vi "Transcriptor LabVIEW to C code Translator 2.vi"(0 "Input":variant=variant("Function Name"=variant(string "Strip Path"), "Input Datatypes"=variant(string[] ["error", "int"]), "Inputs"=variant(string[] ["error in", "x"]), "Node refnum"=variant(refnum<vi> refnum), "Output Datatypes"=variant(string[] ["int"]), "Outputs"=variant(string[] ["a"])), 11 "error in (no error)":errorcluster) -> (4 "Output":variant=variant("Defines"=variant(string[] []), "Includes"=variant(string[] []), "Replaced Code"=variant(string "/* LabVIEW system function 'Strip Path' not found. */")), 15 "error out":errorcluster)   [LabVIEW 2014]
doc: "An example of how to create the Translator to convert the LabVIEW VIs to Arduino C code."
panel:
  out "Outputs":string[](array[string])
  out "Inputs":string[](array[string])
  out "Output Datatypes":string[](array[string])
  out "Input Datatypes":string[](array[string])
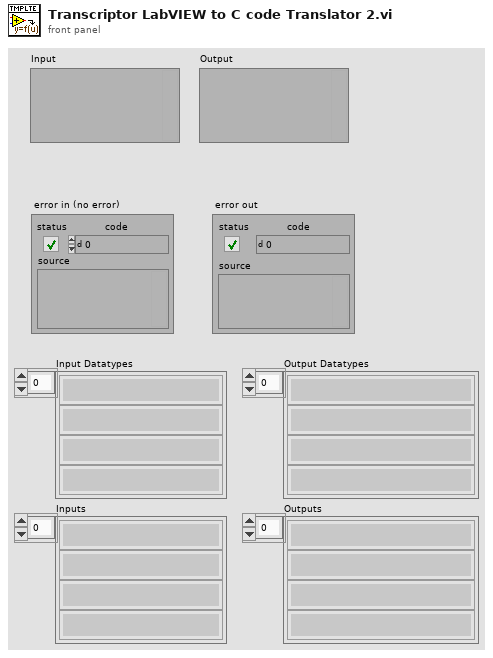
[diagram p1: front panel]
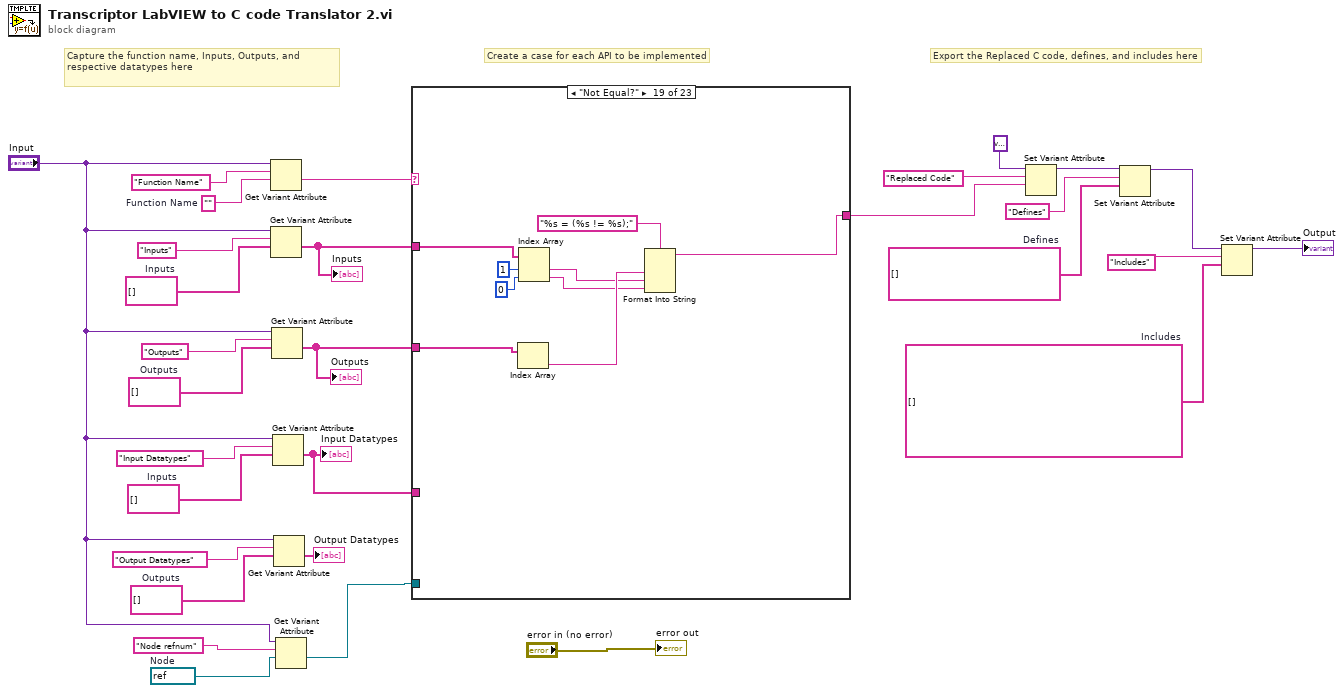
[diagram p0: block diagram]
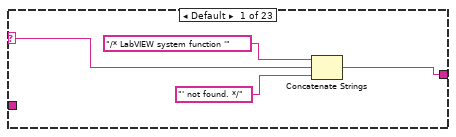
[diagram p2: hidden frame]
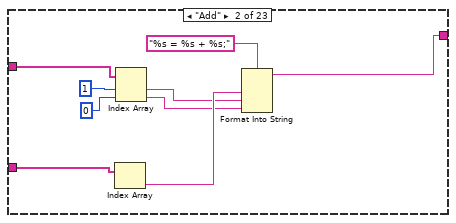
[diagram p3: hidden frame]
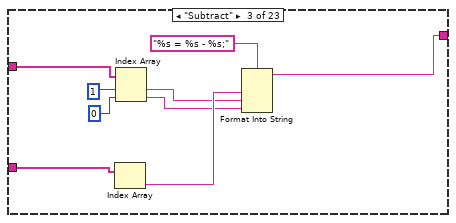
[diagram p4: hidden frame]
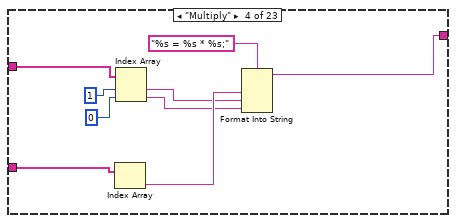
[diagram p5: hidden frame]
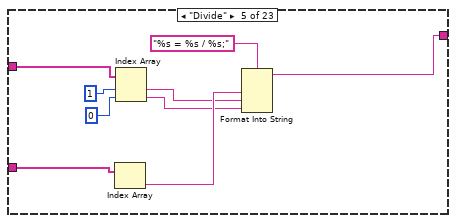
[diagram p6: hidden frame]
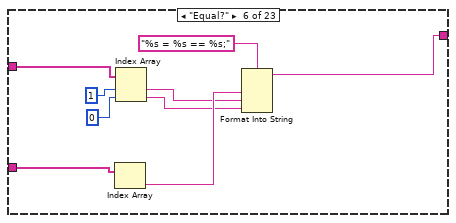
[diagram p7: hidden frame]
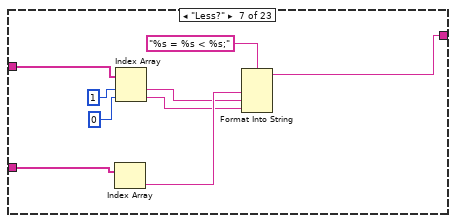
[diagram p8: hidden frame]
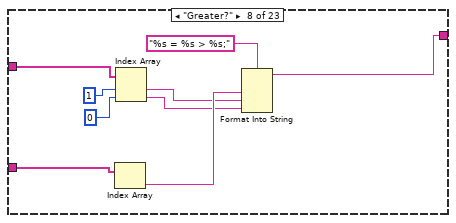
[diagram p9: hidden frame]
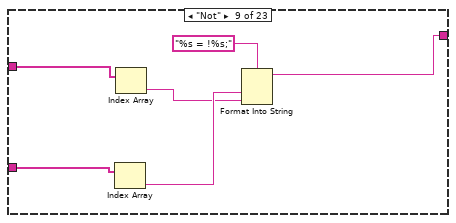
[diagram p10: hidden frame]
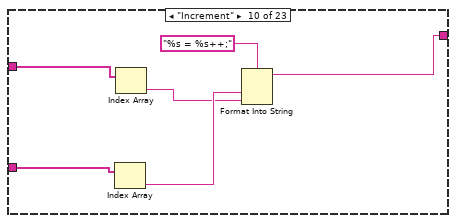
[diagram p11: hidden frame]
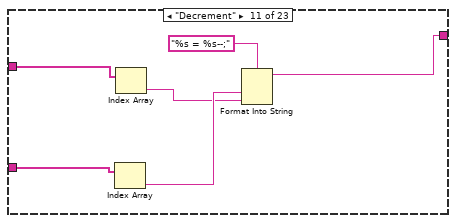
[diagram p12: hidden frame]
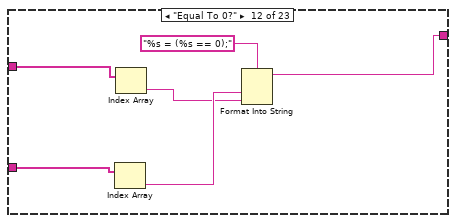
[diagram p13: hidden frame]
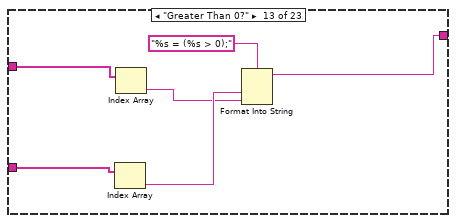
[diagram p14: hidden frame]
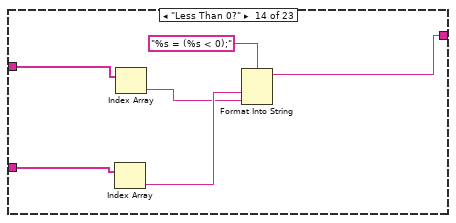
[diagram p15: hidden frame]
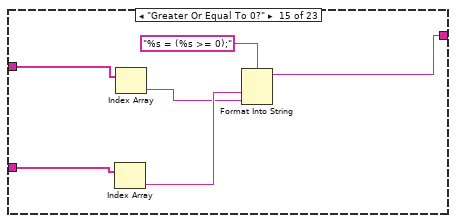
[diagram p16: hidden frame]
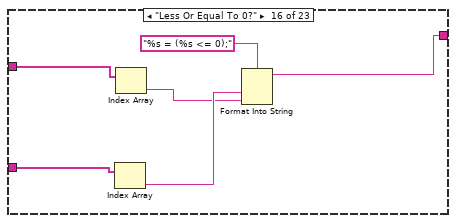
[diagram p17: hidden frame]
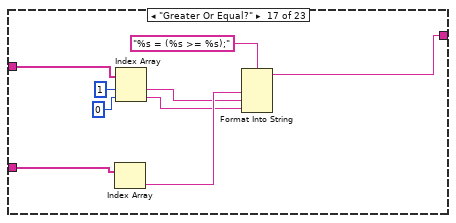
[diagram p18: hidden frame]
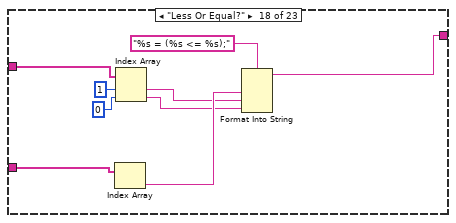
[diagram p19: hidden frame]
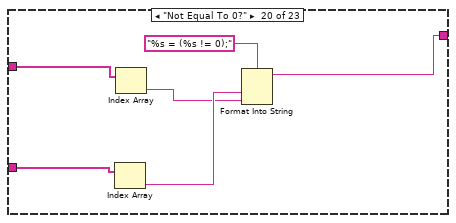
[diagram p20: hidden frame]
diagram:
  w2 = refnum<vi> refnum  # Node
  w6 = string[] []  # Defines
  w15 = string[] []  # Outputs
  w16 = string[] []  # Inputs
  w21 = string[] []  # Includes
  w26 = string[] []  # Outputs
  w27 = string[] []  # Inputs
  w28 = ""  # Function Name
  # "Capture the function name, Inputs, Outputs, and respective datatypes here"
  # "Export the Replaced C code, defines, and includes here"
  # "Create a case for each API to be implemented"
  n1 = Get Variant Attribute(Variant="Input", name="Function Name", default value (empty Variant)=w28) -> (value=w23:string)  [unwired: 1 in, 3 out]
  n2 = Get Variant Attribute(Variant="Input", name="Inputs", default value (empty Variant)=w27) -> (value=w11:string[])  [unwired: 1 in, 3 out]
  "Inputs" <- w11
  n3 = Get Variant Attribute(Variant="Input", name="Outputs", default value (empty Variant)=w26) -> (value=w12:string[])  [unwired: 1 in, 3 out]
  "Outputs" <- w12
  n4 = Get Variant Attribute(Variant="Input", name="Input Datatypes", default value (empty Variant)=w16) -> (value=w5:string[])  [unwired: 1 in, 3 out]
  "Input Datatypes" <- w5
  n5 = Get Variant Attribute(Variant="Input", name="Output Datatypes", default value (empty Variant)=w15) -> (value=→"Output Datatypes":string[])  [unwired: 1 in, 3 out]
  n6 = Get Variant Attribute(Variant="Input", name="Node refnum", default value (empty Variant)=w2) -> (value=w1:refnum<vi>)  [unwired: 1 in, 3 out]
  n7 = case shown="\"Not Equal?\"" w23 {
    selector: w23 -> [w33 _ _ _ _ _ _ _ _ _ _ _ _ _ _ _ _ _ _ _ _ _ _]
    tunnel: [w31 w41 w50 w59 w68 w77 w86 w95 w101 w107 w113 w119 w125 w131 w137 w143 w152 w161 w170 w176 w185 w192 w199] -> w22
    tunnel: w11 -> [_ w43 w52 w61 w70 w79 w88 w97 w103 w109 w115 w121 w127 w133 w139 w145 w154 w163 w172 w178 w187 w194 w201]
    tunnel: w12 -> [_ w40 w49 w58 w67 w76 w85 w94 w100 w106 w112 w118 w124 w130 w136 w142 w151 w160 w169 w175 w184 w191 w198]
    tunnel: w5 -> [_ _ _ _ _ _ _ _ _ _ _ _ _ _ _ _ _ _ _ _ _ _ _]
    tunnel: w1 -> [_ _ _ _ _ _ _ _ _ _ _ _ _ _ _ _ _ _ _ _ _ _ _]
    frame Default {
      n8 = Concatenate Strings("/* LabVIEW system function '", w33, "' not found. */") -> (w31:string)
    }
    frame "Add" {
      n9 = Index Array(array=w40) -> (element=w39:string)  [unwired: 1 in]
      n10 = Index Array(array=w43, index #1=1 ("index"), index #2=0 ("index")) -> (element #1=w38:string, element #2=w37:string)
      n11 = Format Into String(format string="%s = %s + %s;", w39, w38, w37) -> (resulting string=w41:string)  [unwired: 2 in, 1 out]
    }
    frame "Subtract" {
      n12 = Index Array(array=w49) -> (element=w48:string)  [unwired: 1 in]
      n13 = Index Array(array=w52, index #1=1 ("index"), index #2=0 ("index")) -> (element #1=w47:string, element #2=w46:string)
      n14 = Format Into String(format string="%s = %s - %s;", w48, w47, w46) -> (resulting string=w50:string)  [unwired: 2 in, 1 out]
    }
    frame "Multiply" {
      n15 = Index Array(array=w58) -> (element=w57:string)  [unwired: 1 in]
      n16 = Index Array(array=w61, index #1=1 ("index"), index #2=0 ("index")) -> (element #1=w56:string, element #2=w55:string)
      n17 = Format Into String(format string="%s = %s * %s;", w57, w56, w55) -> (resulting string=w59:string)  [unwired: 2 in, 1 out]
    }
    frame "Divide" {
      n18 = Index Array(array=w67) -> (element=w66:string)  [unwired: 1 in]
      n19 = Index Array(array=w70, index #1=1 ("index"), index #2=0 ("index")) -> (element #1=w65:string, element #2=w64:string)
      n20 = Format Into String(format string="%s = %s / %s;", w66, w65, w64) -> (resulting string=w68:string)  [unwired: 2 in, 1 out]
    }
    frame "Equal?" {
      n21 = Index Array(array=w76) -> (element=w75:string)  [unwired: 1 in]
      n22 = Index Array(array=w79, index #1=1 ("index"), index #2=0 ("index")) -> (element #1=w74:string, element #2=w73:string)
      n23 = Format Into String(format string="%s = %s == %s;", w75, w74, w73) -> (resulting string=w77:string)  [unwired: 2 in, 1 out]
    }
    frame "Less?" {
      n24 = Index Array(array=w85) -> (element=w84:string)  [unwired: 1 in]
      n25 = Index Array(array=w88, index #1=1 ("index"), index #2=0 ("index")) -> (element #1=w83:string, element #2=w82:string)
      n26 = Format Into String(format string="%s = %s < %s;", w84, w83, w82) -> (resulting string=w86:string)  [unwired: 2 in, 1 out]
    }
    frame "Greater?" {
      n27 = Index Array(array=w94) -> (element=w93:string)  [unwired: 1 in]
      n28 = Index Array(array=w97, index #1=1 ("index"), index #2=0 ("index")) -> (element #1=w92:string, element #2=w91:string)
      n29 = Format Into String(format string="%s = %s > %s;", w93, w92, w91) -> (resulting string=w95:string)  [unwired: 2 in, 1 out]
    }
    frame "Not" {
      n30 = Index Array(array=w100) -> (element=w99:string)  [unwired: 1 in]
      n31 = Index Array(array=w103) -> (element=w98:string)  [unwired: 1 in]
      n32 = Format Into String(format string="%s = !%s;", w99, w98) -> (resulting string=w101:string)  [unwired: 2 in, 1 out]
    }
    frame "Increment" {
      n33 = Index Array(array=w106) -> (element=w105:string)  [unwired: 1 in]
      n34 = Index Array(array=w109) -> (element=w104:string)  [unwired: 1 in]
      n35 = Format Into String(format string="%s = %s++;", w105, w104) -> (resulting string=w107:string)  [unwired: 2 in, 1 out]
    }
    frame "Decrement" {
      n36 = Index Array(array=w112) -> (element=w111:string)  [unwired: 1 in]
      n37 = Index Array(array=w115) -> (element=w110:string)  [unwired: 1 in]
      n38 = Format Into String(format string="%s = %s--;", w111, w110) -> (resulting string=w113:string)  [unwired: 2 in, 1 out]
    }
    frame "Equal To 0?" {
      n39 = Index Array(array=w118) -> (element=w117:string)  [unwired: 1 in]
      n40 = Index Array(array=w121) -> (element=w116:string)  [unwired: 1 in]
      n41 = Format Into String(format string="%s = (%s == 0);", w117, w116) -> (resulting string=w119:string)  [unwired: 2 in, 1 out]
    }
    frame "Greater Than 0?" {
      n42 = Index Array(array=w124) -> (element=w123:string)  [unwired: 1 in]
      n43 = Index Array(array=w127) -> (element=w122:string)  [unwired: 1 in]
      n44 = Format Into String(format string="%s = (%s > 0);", w123, w122) -> (resulting string=w125:string)  [unwired: 2 in, 1 out]
    }
    frame "Less Than 0?" {
      n45 = Index Array(array=w130) -> (element=w129:string)  [unwired: 1 in]
      n46 = Index Array(array=w133) -> (element=w128:string)  [unwired: 1 in]
      n47 = Format Into String(format string="%s = (%s < 0);", w129, w128) -> (resulting string=w131:string)  [unwired: 2 in, 1 out]
    }
    frame "Greater Or Equal To 0?" {
      n48 = Index Array(array=w136) -> (element=w135:string)  [unwired: 1 in]
      n49 = Index Array(array=w139) -> (element=w134:string)  [unwired: 1 in]
      n50 = Format Into String(format string="%s = (%s >= 0);", w135, w134) -> (resulting string=w137:string)  [unwired: 2 in, 1 out]
    }
    frame "Less Or Equal To 0?" {
      n51 = Index Array(array=w142) -> (element=w141:string)  [unwired: 1 in]
      n52 = Index Array(array=w145) -> (element=w140:string)  [unwired: 1 in]
      n53 = Format Into String(format string="%s = (%s <= 0);", w141, w140) -> (resulting string=w143:string)  [unwired: 2 in, 1 out]
    }
    frame "Greater Or Equal?" {
      n54 = Index Array(array=w151) -> (element=w150:string)  [unwired: 1 in]
      n55 = Index Array(array=w154, index #1=1 ("index"), index #2=0 ("index")) -> (element #1=w149:string, element #2=w146:string)
      n56 = Format Into String(format string="%s = (%s >= %s);", w150, w149, w146) -> (resulting string=w152:string)  [unwired: 2 in, 1 out]
    }
    frame "Less Or Equal?" {
      n57 = Index Array(array=w160) -> (element=w159:string)  [unwired: 1 in]
      n58 = Index Array(array=w163, index #1=1 ("index"), index #2=0 ("index")) -> (element #1=w158:string, element #2=w155:string)
      n59 = Format Into String(format string="%s = (%s <= %s);", w159, w158, w155) -> (resulting string=w161:string)  [unwired: 2 in, 1 out]
    }
    frame "Not Equal?" {
      n60 = Index Array(array=w169) -> (element=w168:string)  [unwired: 1 in]
      n61 = Index Array(array=w172, index #1=1 ("index"), index #2=0 ("index")) -> (element #1=w167:string, element #2=w164:string)
      n62 = Format Into String(format string="%s = (%s != %s);", w168, w167, w164) -> (resulting string=w170:string)  [unwired: 2 in, 1 out]
    }
    frame "Not Equal To 0?" {
      n63 = Index Array(array=w175) -> (element=w174:string)  [unwired: 1 in]
      n64 = Index Array(array=w178) -> (element=w173:string)  [unwired: 1 in]
      n65 = Format Into String(format string="%s = (%s != 0);", w174, w173) -> (resulting string=w176:string)  [unwired: 2 in, 1 out]
    }
    frame "And" {
      n66 = Index Array(array=w184) -> (element=w183:string)  [unwired: 1 in]
      n67 = Index Array(array=w187, index #1=1 ("index"), index #2=0 ("index")) -> (element #1=w182:string, element #2=w181:string)
      n68 = Format Into String(format string="%s = %s AND %s;", w183, w182, w181) -> (resulting string=w185:string)  [unwired: 2 in, 1 out]
    }
    frame "Or" {
      n69 = Index Array(array=w191) -> (element=w190:string)  [unwired: 1 in]
      n70 = Index Array(array=w194) -> (element #1=w189:string, element #2=w188:string)  [unwired: 2 in]
      n71 = Format Into String(format string="%s = %s OR %s;", w190, w189, w188) -> (resulting string=w192:string)  [unwired: 2 in, 1 out]
    }
    frame "Exclusive Or" {
      n72 = Index Array(array=w198) -> (element=w197:string)  [unwired: 1 in]
      n73 = Index Array(array=w201) -> (element #1=w196:string, element #2=w195:string)  [unwired: 2 in]
      n74 = Format Into String(format string="%s = %s XOR %s;", w197, w196, w195) -> (resulting string=w199:string)  [unwired: 2 in, 1 out]
    }
  }
  n75 = Set Variant Attribute(Variant=variant ("variant"), name="Replaced Code", value=w22) -> (Variant out=w9:variant)  [unwired: 1 in, 2 out]
  n76 = Set Variant Attribute(Variant=w9, name="Defines", value=w6) -> (Variant out=w8:variant)  [unwired: 1 in, 2 out]
  n77 = Set Variant Attribute(Variant=w8, name="Includes", value=w21) -> (Variant out=→"Output":variant)  [unwired: 1 in, 2 out]
  "error out" <- "error in (no error)"
